vi "xyGraphInputs.vi"() -> ()   [LabVIEW 2014]
panel:
  in  "Number of Plots":i32(slide) scale=0.0..10.0
  out "XY Graph 6 (Multiple Plots, Array of Clusters of Arrays of Complex Values)":cluster{cdb[]}[](graph)
  out "XY Graph 5 (Multiple Plots, Array of Clusters)":cluster{cluster{dbl, dbl}[]}[](graph)
  out "XY Graph 4 (Multiple Plots, Array of Clusters of Arrays)":cluster{dbl[], dbl[]}[](graph)
  in  "Number of Graph Points":i32(slide) scale=0.0..100.0
  out "XY Graph 3 (Single Plot, Array of Complex Values)":cdb[](graph)
  out "XY Graph 2 (Single Plot, Array of Clusters)":cluster{"X":dbl, "Y":dbl}[](graph)
  out "XY Graph 1 (Single Plot, Cluster of Arrays)":cluster{dbl[], dbl[]}(graph)
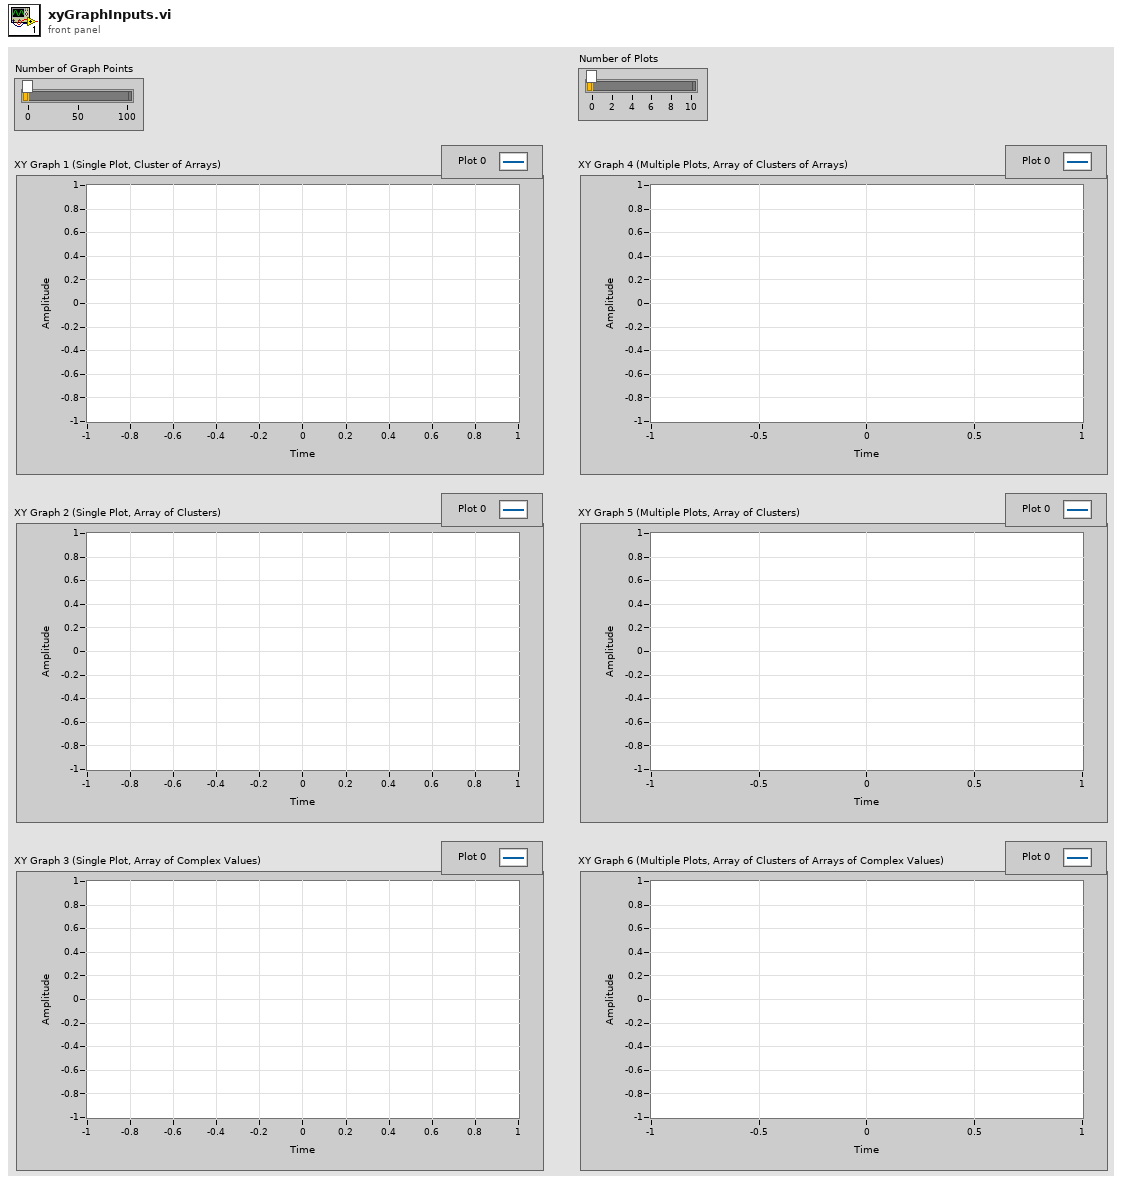
[diagram p1: front panel]
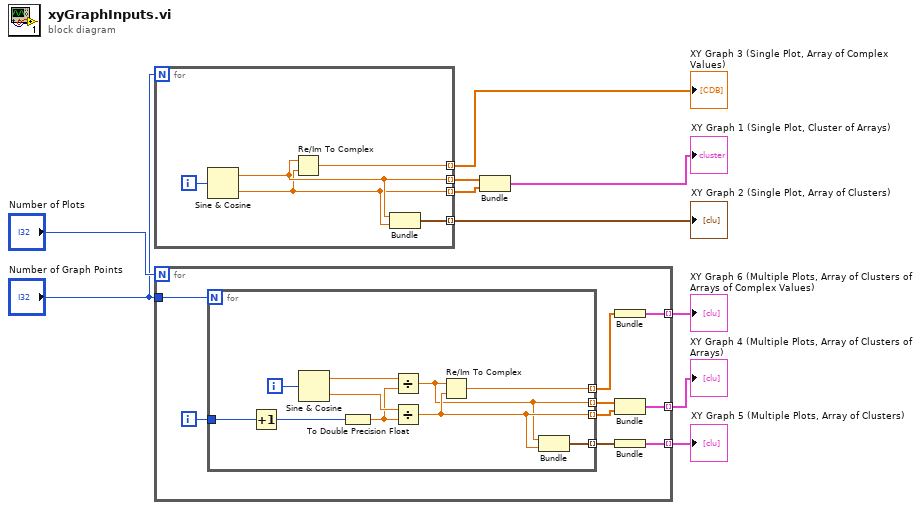
[diagram p0: block diagram]
diagram:
  n1 = for {
    N: "Number of Graph Points" -> [_]
    tunnel: [w14] -> w10 mode=indexing
    tunnel: [w13] -> w9 mode=indexing
    tunnel: [w12] -> w8 mode=indexing
    tunnel: [w11] -> w6 mode=indexing
    i -> [w15]
    n2 = Sine & Cosine(0:w15) -> (1:w13:dbl, 2:w12:dbl)
    n3 = Re/Im To Complex(1:w12, 2:w13) -> (0:w14:cdb)
    n4 = Bundle "Bundle"(w13, w12) -> (w11:cluster{dbl, dbl})  [unwired: 1 in]
  }
  "XY Graph 2 (Single Plot, Array of Clusters)" <- w6
  "XY Graph 3 (Single Plot, Array of Complex Values)" <- w10
  n5 = for {
    N: "Number of Plots" -> [_]
    tunnel: "Number of Graph Points" -> [w24]
    tunnel: [w19] -> w5 mode=indexing
    tunnel: [w21] -> w4 mode=indexing
    tunnel: [w17] -> w3 mode=indexing
    i -> [w16]
    n6 = for {
      N: w24 -> [_]
      tunnel: [w34] -> w20 mode=indexing
      tunnel: [w28] -> w23 mode=indexing
      tunnel: [w30] -> w22 mode=indexing
      tunnel: [w31] -> w18 mode=indexing
      tunnel: w16 -> [w25]
      i -> [w29]
      n7 = Increment(x=w25) -> (x+1=w26:i32)
      n8 = Sine & Cosine(0:w29) -> (1:w33:dbl, 2:w32:dbl)
      n9 = To Double Precision Float(number=w26) -> (double precision float=w27:dbl)
      n10 = Divide(x=w33, y=w27) -> (x/y=w28:dbl)
      n11 = Divide(x=w32, y=w27) -> (x/y=w30:dbl)
      n12 = Re/Im To Complex(1:w30, 2:w28) -> (0:w34:cdb)
      n13 = Bundle "Bundle"(w28, w30) -> (w31:cluster{dbl, dbl})  [unwired: 1 in]
    }
    n14 = Bundle "Bundle"(w20) -> (w19:cluster{cdb[]})  [unwired: 1 in]
    n15 = Bundle "Bundle"(w23, w22) -> (w21:cluster{dbl[], dbl[]})  [unwired: 1 in]
    n16 = Bundle "Bundle"(w18) -> (w17:cluster{cluster{dbl, dbl}[]})  [unwired: 1 in]
  }
  "XY Graph 4 (Multiple Plots, Array of Clusters of Arrays)" <- w4
  "XY Graph 5 (Multiple Plots, Array of Clusters)" <- w3
  "XY Graph 6 (Multiple Plots, Array of Clusters of Arrays of Complex Values)" <- w5
  n17 = Bundle "Bundle"(w9, w8) -> (→"XY Graph 1 (Single Plot, Cluster of Arrays)":cluster{dbl[], dbl[]})  [unwired: 1 in]
